vi "SensorConfigToJSON.vi"(6 "StreamType":T1, 8 "ErrorIn":errorcluster, 10 "SensorConfig":T2={"AccelFSRange"=enum."2G", "GyroFSRange"=enum."250DPS", "ODR"=enum."10HZ", "AccelDLPF"=enum."5HZ", "GyroDLPF"=enum."5HZ", "InterruptPinMode"=enum."OPEN_DRAIN_FALLING_EDGE", "InterruptMode"=enum."DATA_RDY", "Resolution"=4} {"Resolution" min=4 max=16 step=1}, 11 "JSONIn":refnum<class "JSON Object.lvclass">) -> (0 "ErrorOut":errorcluster, 2 "JSONSensorConfig":string, 3 "JSONOut":refnum<class "JSON Object.lvclass">)   [LabVIEW 2016]
uses:
  <vilib>/addons/JSON API/JSON Object/JSON Object.lvclass
  D:/Programy/National Instruments/LabVIEW 2016/vi.lib/addons/JSON API/JSON Value/JSON Value.lvclass
  FallSensor/ConfigureDevice/CDSensorConfiguration.ctl
  FallSensor/ConfigureDevice/CDAccelFSRange.ctl
  FallSensor/ConfigureDevice/CDGyroFSRange.ctl
  FallSensor/ConfigureDevice/CDOutputDataRate.ctl
  FallSensor/ConfigureDevice/CDAccelDLPF.ctl
  FallSensor/ConfigureDevice/CDGyroDLPF.ctl
  FallSensor/ConfigureDevice/CDInterruptPinMode.ctl
  FallSensor/ConfigureDevice/CDInterruptMode.ctl
  JSONStreamType.ctl
  <vilib>/addons/JSON API/JSON Object/Set Object Item by name.vi
  <vilib>/addons/JSON API/JSON Value/Get as JSON string.vi
  <vilib>/addons/JSON API/JSON Scalar/JSON Scalar.lvclass
  <vilib>/addons/JSON API/JSON Scalar/Set String.vi
  <vilib>/addons/JSON API/JSON Scalar/Set U32.vi
  <vilib>/addons/JSON API/JSON Value/Get as JSON string (pretty).vi
  <vilib>/addons/JSON API/JSON Value/Get Item by name array.vi
  <vilib>/addons/JSON API/JSON Value/JSON Value.lvclass
  <vilib>/addons/JSON API/Get Polymorphic/JSON GetSet.lvlib
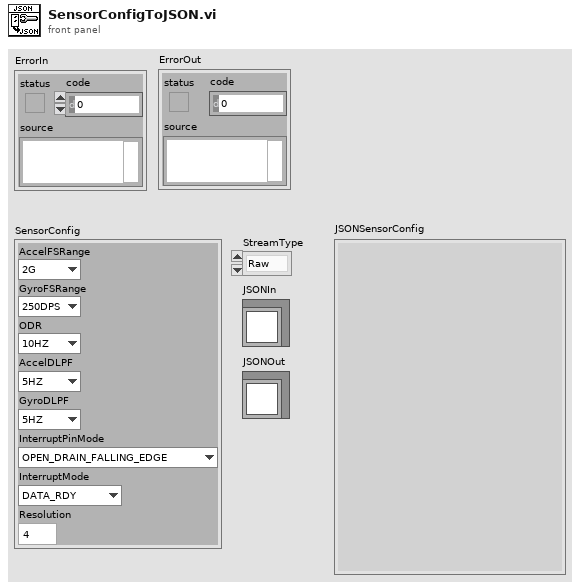
[diagram p1: front panel]
types:
  T1 = typedef "JSONStreamType.ctl" = enum16{"Raw", "Pretty"}
  T2 = typedef "CDSensorConfiguration.ctl" = cluster{"AccelFSRange":T3, "GyroFSRange":T4, "ODR":T5, "AccelDLPF":T6, "GyroDLPF":T7, "InterruptPinMode":T8, "InterruptMode":T9, "Resolution":u32}
  T3 = typedef "CDAccelFSRange.ctl" = enum16{"2G", "4G", "8G", "16G"}
  T4 = typedef "CDGyroFSRange.ctl" = enum16{"250DPS", "500DPS", "1000DPS", "2000DPS"}
  T5 = typedef "CDOutputDataRate.ctl" = enum16{"10HZ", "20HZ", "40HZ", "50HZ", "100HZ", "200HZ", "500HZ", "1000HZ"}
  T6 = typedef "CDAccelDLPF.ctl" = enum16{"5HZ", "10HZ", "20HZ", "41HZ", "92HZ", "184HZ", "460HZ"}
  T7 = typedef "CDGyroDLPF.ctl" = enum16{"5HZ", "10HZ", "20HZ", "41HZ", "92HZ", "184HZ"}
  T8 = typedef "CDInterruptPinMode.ctl" = enum16{"OPEN_DRAIN_FALLING_EDGE"}
  T9 = typedef "CDInterruptMode.ctl" = enum16{"DATA_RDY"}
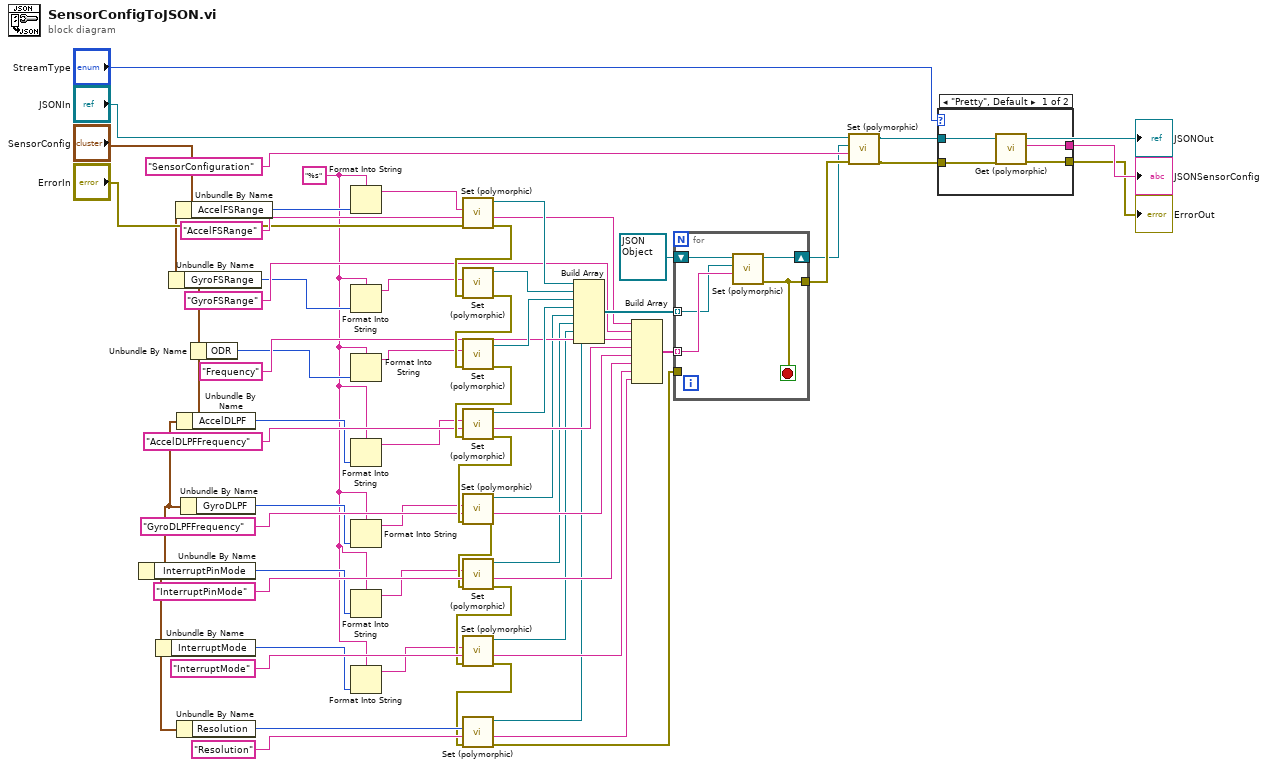
[diagram p0: block diagram]
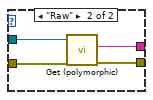
[diagram p2: hidden frame]
diagram:
  w1 = "%s"
  n1 = Unbundle By Name("SensorConfig") -> ("InterruptPinMode"=w6:T8)
  n2 = Unbundle By Name("SensorConfig") -> ("InterruptMode"=w5:T9)
  n3 = Unbundle By Name("SensorConfig") -> ("GyroFSRange"=w13:T4)
  n4 = Unbundle By Name("SensorConfig") -> ("AccelFSRange"=w15:T3)
  n5 = Unbundle By Name("SensorConfig") -> ("AccelDLPF"=w9:T6)
  n6 = Unbundle By Name("SensorConfig") -> ("Resolution"=w21:u32)
  n7 = Unbundle By Name("SensorConfig") -> ("GyroDLPF"=w7:T7)
  n8 = Unbundle By Name("SensorConfig") -> ("ODR"=w12:T5)
  n9 = Format Into String(format string=w1, w15) -> (resulting string=w14:string)  [unwired: 2 in, 1 out]
  n10 = Format Into String(format string=w1, w13) -> (resulting string=w10:string)  [unwired: 2 in, 1 out]
  n11 = Format Into String(format string=w1, w12) -> (resulting string=w11:string)  [unwired: 2 in, 1 out]
  n12 = Format Into String(format string=w1, w9) -> (resulting string=w8:string)  [unwired: 2 in, 1 out]
  n13 = Format Into String(format string=w1, w7) -> (resulting string=w4:string)  [unwired: 2 in, 1 out]
  n14 = Format Into String(format string=w1, w6) -> (resulting string=w3:string)  [unwired: 2 in, 1 out]
  n15 = Format Into String(format string=w1, w5) -> (resulting string=w2:string)  [unwired: 2 in, 1 out]
  n16 = call-poly <vilib>:"Set (polymorphic).vi"("error in (no error)"="ErrorIn", "String"=w14) -> ("error out"=w50:errorcluster, "JSON Scalar out"=w54:refnum<class "JSON Scalar.lvclass">)  [unwired: 8 in]
  n17 = call-poly <vilib>:"Set (polymorphic).vi"("error in (no error)"=w50, "String"=w10) -> ("error out"=w49:errorcluster, "JSON Scalar out"=w53:refnum<class "JSON Scalar.lvclass">)  [unwired: 8 in]
  n18 = call-poly <vilib>:"Set (polymorphic).vi"("error in (no error)"=w49, "String"=w11) -> ("error out"=w48:errorcluster, "JSON Scalar out"=w52:refnum<class "JSON Scalar.lvclass">)  [unwired: 8 in]
  n19 = call-poly <vilib>:"Set (polymorphic).vi"("error in (no error)"=w48, "String"=w8) -> ("error out"=w30:errorcluster, "JSON Scalar out"=w51:refnum<class "JSON Scalar.lvclass">)  [unwired: 8 in]
  n20 = call-poly <vilib>:"Set (polymorphic).vi"("error in (no error)"=w30, "String"=w4) -> ("error out"=w25:errorcluster, "JSON Scalar out"=w28:refnum<class "JSON Scalar.lvclass">)  [unwired: 8 in]
  n21 = call-poly <vilib>:"Set (polymorphic).vi"("error in (no error)"=w25, "String"=w3) -> ("error out"=w22:errorcluster, "JSON Scalar out"=w26:refnum<class "JSON Scalar.lvclass">)  [unwired: 8 in]
  n22 = call-poly <vilib>:"Set (polymorphic).vi"("error in (no error)"=w22, "String"=w2) -> ("error out"=w16:errorcluster, "JSON Scalar out"=w23:refnum<class "JSON Scalar.lvclass">)  [unwired: 8 in]
  n23 = call-poly <vilib>:"Set (polymorphic).vi"("error in (no error)"=w16, "Numeric"=w21) -> ("error out"=w17:errorcluster, "JSON Scalar out"=w19:refnum<class "JSON Scalar.lvclass">)  [unwired: 8 in]
  n24 = Build Array(w54, w53, w52, w51, w28, w26, w23, w19) -> (w46:refnum<class "JSON Scalar.lvclass">[])
  n25 = Build Array("AccelFSRange" ("name"), "GyroFSRange" ("name"), "Frequency" ("name"), "AccelDLPFFrequency" ("name"), "GyroDLPFFrequency" ("name"), "InterruptPinMode" ("name"), "InterruptMode" ("name"), "Resolution" ("name")) -> (w41:string[])
  n26 = for {
    shift-right: [w56] -> w38
    shift-left: refnum<class "JSON Object.lvclass"> refnum ("JSON Object out") -> [w59]
    tunnel: w46 -> [w57] mode=indexing
    tunnel: w41 -> [w58] mode=indexing
    tunnel: [w55] -> w39
    tunnel: w17 -> [_]
    stop <- w55 stop-if-true
    n27 = call-poly <vilib>:"Set (polymorphic).vi"("name"=w58, "Value"=w57, "JSON Object in"=w59) -> ("error out"=w55:errorcluster, "JSON Object out"=w56:refnum<class "JSON Object.lvclass">)  [unwired: 6 in, 1 out]
  }
  n28 = call-poly <vilib>:"Set (polymorphic).vi"("error in (no error)"=w39, "name"="SensorConfiguration", "Value"=w38, "JSON Object in"="JSONIn") -> ("error out"=w37:errorcluster, "JSON Object out"=w36:refnum<class "JSON Object.lvclass">)  [unwired: 5 in, 1 out]
  "JSONOut" <- w36
  n29 = case shown="\"Pretty\", Default" "StreamType" {
    tunnel: w37 -> [w63 w67]
    tunnel: w36 -> [w62 w66]
    tunnel: [w61 w65] -> w33
    tunnel: [w60 w64] -> w32
    frame "Pretty", Default {
      n30 = call-poly <vilib>:"Get (polymorphic).vi"("error in (no error)"=w63, "JSON Value in"=w62) -> ("error out"=w60:errorcluster, "<JSON>"=w61:string)  [unwired: 8 in]
    }
    frame "Raw" {
      n31 = call-poly <vilib>:"Get (polymorphic).vi"("error in (no error)"=w67, "JSON Value in"=w66) -> ("error out"=w64:errorcluster, "<JSON>"=w65:string)  [unwired: 8 in]
    }
  }
  "ErrorOut" <- w32
  "JSONSensorConfig" <- w33
